vi "Parse Error.vi"(8 "error in (no error)":errorcluster, 11 "JSON Value in":refnum<class "JSON Value.lvclass">) -> (0 "error out":errorcluster, 3 "JSON Value out":refnum<class "JSON Value.lvclass">)   [LabVIEW 2011, in "JSON Value.lvclass"]
uses:
  JSON Value.lvclass
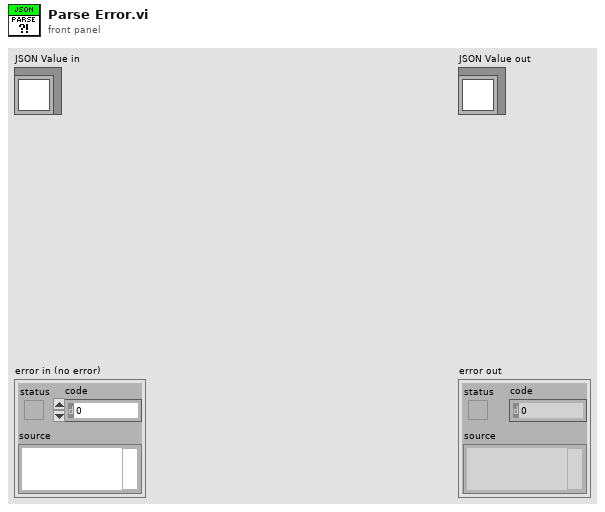
[diagram p1: front panel]
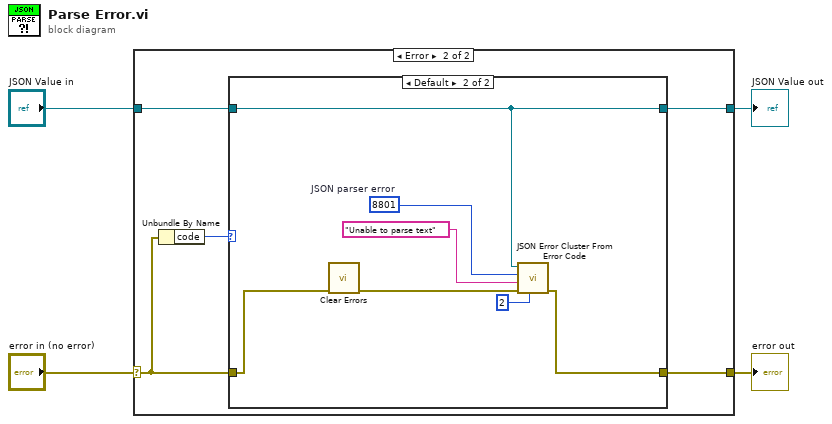
[diagram p0: block diagram]
diagram:
  n1 = case shown="Error" "error in (no error)" {
    selector: "error in (no error)" -> [w6 w10]
    tunnel: [w6 w11] -> w3
    tunnel: [w5 w7] -> w1
    tunnel: "JSON Value in" -> [w5 w8]
    frame No Error {
    }
    frame Error {
      n2 = Unbundle By Name(w10) -> ("code"=w9:i32)
      n3 = case shown="Default" w9 {
        tunnel: [w12 w18] -> w11
        tunnel: w8 -> [w13 w17]
        tunnel: w10 -> [w12 w19]
        tunnel: [w13 w17] -> w7
        frame 8801..8810 {
          # "Already reporting a JSON error from a lower level"
        }
        frame Default {
          w16 = 8801  # JSON parser error
          n4 = call <vilib>:"Clear Errors.vi"("error in (no error)"=w19) -> ("error out"=w14:errorcluster)  [unwired: 6 in]
          n5 = call "JSON Error Cluster From Error Code.vi"("VI depth (1)"=2, "error in (no error)"=w14, "Error message"="Unable to parse text", "JSON error code"=w16, "JSON Value in"=w17) -> ("error out"=w18:errorcluster)  [unwired: 5 in, 1 out]
        }
      }
    }
  }
  "error out" <- w3
  "JSON Value out" <- w1
